vi "niFpga wdp fft DIT 2spc.vi"(0 "real data in":fxp<+/-,8,1>[](array[numeric])=[0.0, 0.0], 5 "imaginary data in":fxp<+/-,8,1>[](array[numeric])=[0.0, 0.0], 9 "input frame start":bool, 12 "enable":bool) -> (3 "data indices":u16[](array[numeric]), 4 "real data out":fxp<+,8,1>[](array[numeric]), 6 "imaginary data out":fxp<+,8,1>[](array[numeric]), 10 "output valid":bool, 14 "ready for frame":bool, 15 "output frame start":bool)   [LabVIEW 2017]
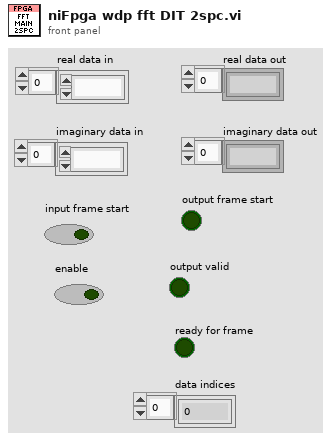
[diagram p1: front panel]
types:
  T1 = cluster{"internal input type":fxp<+/-,8,1>, "internal input type":fxp<+/-,8,1>}
  T2 = cluster{"twiddle factor type":fxp<+/-,16,2>, "twiddle factor type":fxp<+/-,16,2>}[]
  T3 = cluster{"x-y":fxp<+/-,19,12>, "x-y":fxp<+/-,19,12>}
  T4 = cluster{"x+y":fxp<+/-,19,12>, "x+y":fxp<+/-,19,12>}
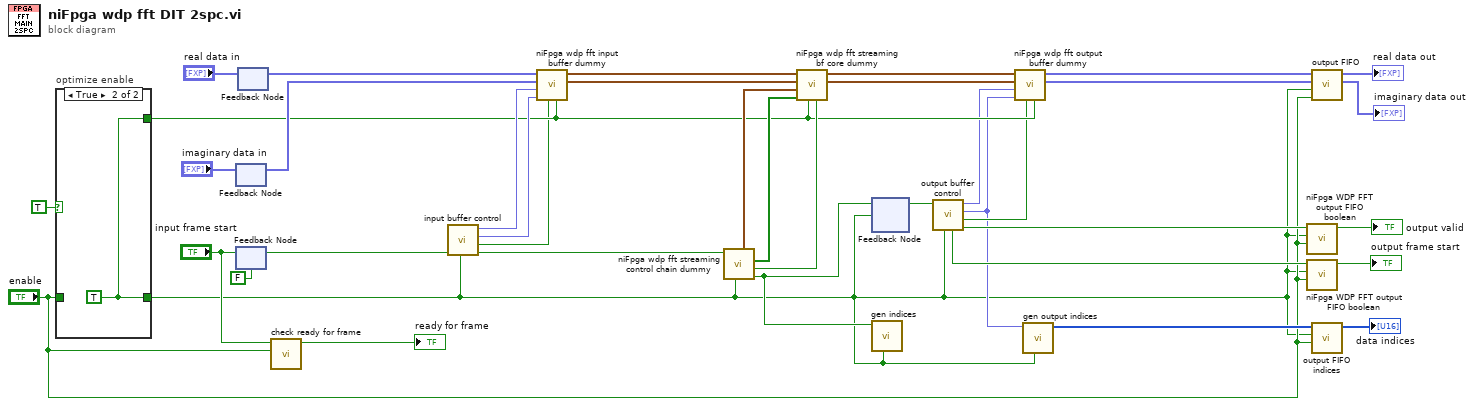
[diagram p0: block diagram]
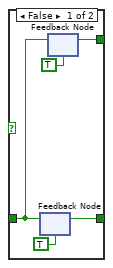
[diagram p2: hidden frame]
diagram:
  n1 = case "optimize enable" shown="True" TRUE {
    tunnel: "enable" -> [w41 _]
    tunnel: [w40 w44] -> w1
    tunnel: [w39 w44] -> w19
    frame False {
      n2 = feedback #1(TRUE ("enable")) -> (w40:bool)
      n3 = feedback-in #1(w41) -> ()
      n4 = feedback #2(TRUE ("enable")) -> (w39:bool)
      n5 = feedback-in #2(w41) -> ()
    }
    frame True {
      w44 = TRUE
    }
  }
  n6 = feedback #3() -> (w24:fxp<+/-,8,1>[])  [unwired: 1 in]
  n7 = feedback-in #3("imaginary data in") -> ()
  n8 = feedback #4(FALSE ("enable")) -> (w33:bool)
  n9 = feedback-in #4("input frame start") -> ()
  n10 = feedback-in #5("real data in") -> ()
  n11 = feedback #5() -> (w25:fxp<+/-,8,1>[])  [unwired: 1 in]
  n12 = call "check ready for frame"("enable"="enable", "frame start in"="input frame start") -> ("ready for frame"=→"ready for frame":bool)  [unwired: 9 in]
  n13 = call "input buffer control"("enable"=w1, "frame start in"=w33) -> ("frame start out"=w31:bool, "write memory 2?"=w13:bool, "read index"=w20:fxp<+,9,9>, "write index"=w21:fxp<+,8,8>)  [unwired: 6 in]
  n14 = call <vilib>:"niFpga wdp fft input buffer dummy.vi"("enable"=w19, "write memory 2?"=w13, "read index"=w20, "write index"=w21, "data in im"=w24, "data in re"=w25) -> ("data out 1"=w22:T1, "data out 0"=w23:T1)  [unwired: 4 in]
  n15 = call <vilib>:"niFpga wdp fft streaming control chain dummy.vi"("enable"=w1, "input frame start"=w31) -> ("frame start"=w2:bool, "index=0?"=w28:bool, "switch"=w29:bool[], "twiddle factors"=w30:T2)  [unwired: 5 in, 1 out]
  n16 = call <vilib>:"niFpga wdp fft streaming bf core dummy.vi"("index=0?"=w28, "enable"=w19, "switch"=w29, "twiddle factors"=w30, "data in 1"=w22, "data in 0"=w23) -> ("data out 1"=w26:T3, "data out 0"=w27:T4)  [unwired: 4 in]
  n17 = feedback #6 ("delay")() -> (w3:bool)  [unwired: 1 in]
  n18 = feedback-in #6(w2, w1) -> ()
  n19 = call "gen indices"("enable"=w1, "frame start"=w2) -> ()  [unwired: 8 in, 2 out]
  n20 = call "output buffer control"("enable"=w1, "frame start"=w3) -> ("output valid?"=w9:bool, "memory switch"=w7:bool, "read index"=w5:fxp<+,4,4>, "write index"=w8:fxp<+,9,9>, "frame start?"=w10:bool)  [unwired: 5 in]
  n21 = call <vilib>:"niFpga wdp fft output buffer dummy.vi"("enable"=w19, "memory switch"=w7, "read index"=w5, "write index"=w8, "data in 1"=w26, "data in 0"=w27) -> ("data out im"=w16:fxp<+/-,32,16>[], "data out re"=w17:fxp<+/-,32,16>[])  [unwired: 4 in]
  n22 = call "gen output indices"("enable"=w1, "index"=w5) -> ("data indices"=w6:u16[])  [unwired: 9 in]
  n23 = call <vilib>:"niFpga WDP FFT output FIFO boolean.vi"("enable"="enable", "enable with delay"=w1, "boolean in"=w9) -> ("boolean out"=→"output valid":bool)  [unwired: 8 in]
  n24 = call <vilib>:"niFpga WDP FFT output FIFO boolean.vi"("enable"="enable", "enable with delay"=w1, "boolean in"=w10) -> ("boolean out"=→"output frame start":bool)  [unwired: 8 in]
  n25 = call "output FIFO"("enable"="enable", "enable with delay"=w1, "data in 1"=w16, "data in 0"=w17) -> ("data out 1"=→"imaginary data out":fxp<+,8,1>[], "data out 0"=→"real data out":fxp<+,8,1>[])  [unwired: 6 in]
  n26 = call "output FIFO indices"("enable"="enable", "enable with delay"=w1, "data in"=w6) -> ("data out"=→"data indices":u16[])  [unwired: 8 in]
